vi "Refilderefrescos.vi"() -> ()   [LabVIEW 2020]
uses:
  <vilib>/LabVIEW Interface for Arduino/Type Defs/Board Type.ctl
  <vilib>/LabVIEW Interface for Arduino/Type Defs/Pin Mode.ctl
  <vilib>/LabVIEW Interface for Arduino/LabVIEW Interface for Arduino.lvlib
panel:
  out "Number of bottles made":dbl
  out "¿Lleno?":dbl(slide) scale=0.0..5.0
  out "BomC1":bool
  out "BomC2":bool
  out "BomC3":bool
  out "BomC4":bool
  out "BomT4":bool
  out "BomT3":bool
  out "BomT2":bool
  out "BomT1":bool
  out "Información Adicional":string
  out "Detección":string
  out "Paro":bool
  out "Marcha":bool
  in  "Total Stop":bool
  in  "VISA resource":refnum<visa-resource-name>
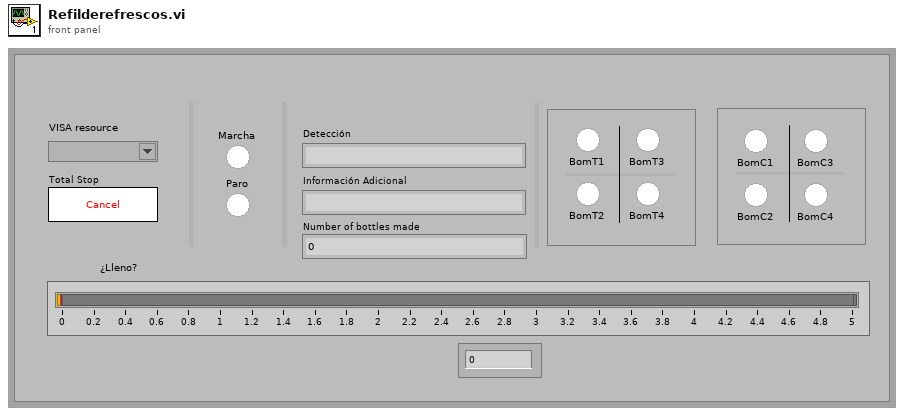
[diagram p1: front panel]
types:
  T1 = typedef "LabVIEW Interface for Arduino.lvlib/Pin Mode.ctl" = enum8{"Input", "Output"}
  T2 = typedef "LabVIEW Interface for Arduino.lvlib/Board Type.ctl" = enum16{"Uno", "Dimuelanove w/Atmega 328", "Mega 2560"}
  T3 = typedef "LabVIEW Interface for Arduino.lvlib/Arduino Resource.ctl" = cluster{"VISA resource":refnum<visa-resource-name>, "Board Type":T2, "Connection Type":enum8{"USB / Serial"}, "Bytes Per Packet (15)":u8}
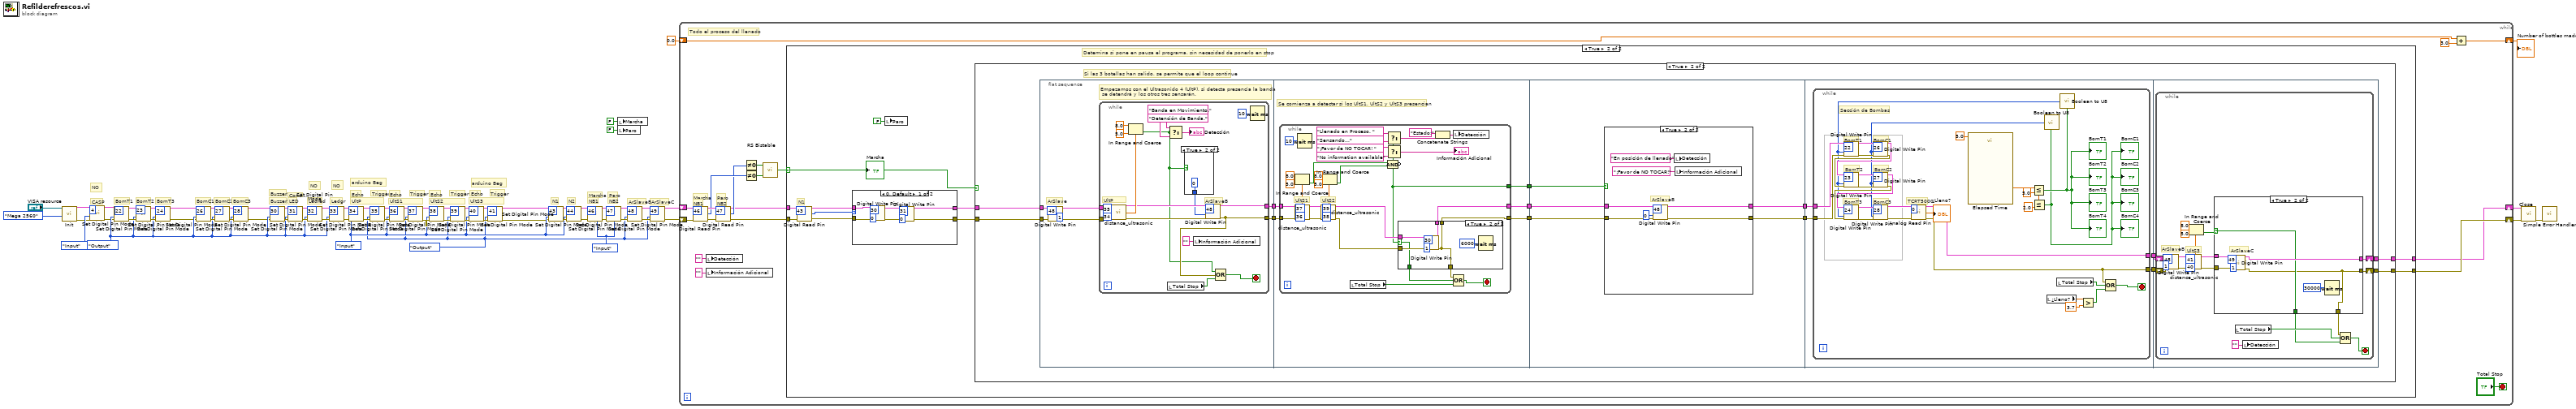
[diagram p0: block diagram]
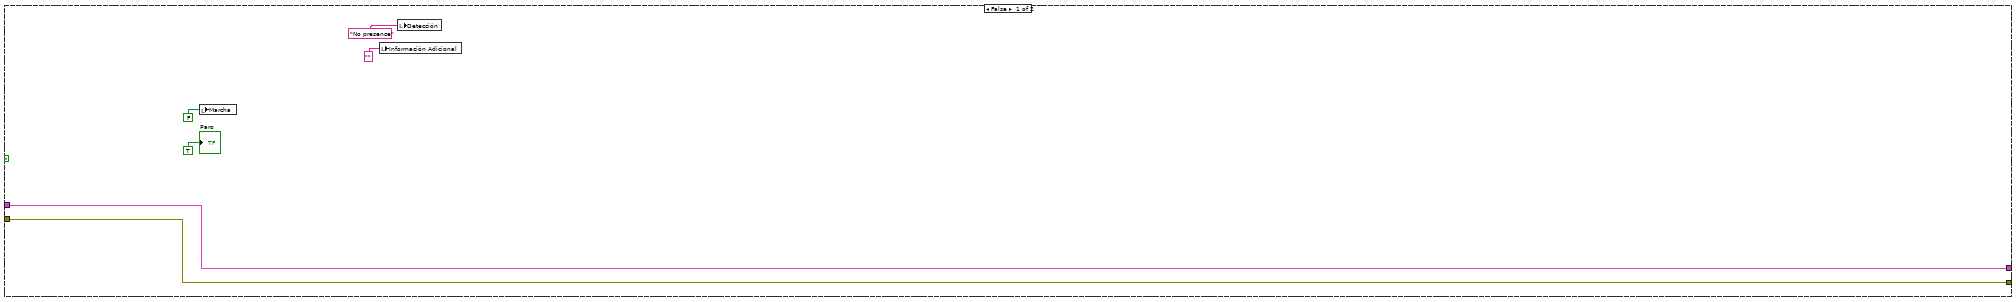
[diagram p2: hidden frame]
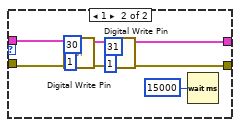
[diagram p3: hidden frame]
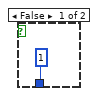
[diagram p5: hidden frame]
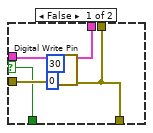
[diagram p6: hidden frame]
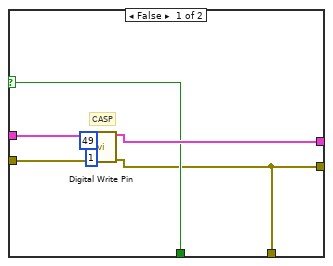
[diagram p8: hidden frame]
diagram:
  w26 = Pin_Mode."Input" ("Pin Mode (Input)")
  w21 = Pin_Mode."Output" ("Pin Mode (Input)")
  w31 = Pin_Mode."Input" ("Pin Mode (Input)")
  w65 = Pin_Mode."Output" ("Pin Mode (Input)")
  # "arduino Beg"
  # "arduino Beg"
  # "NO"
  # "NO"
  # "NO"
  # "Buzzer1"
  # "Condensado"
  # "ArSlaveC"
  # "CASP"
  # "ArSlaveB"
  # "Trigger"
  # "Echo"
  # "Trigger"
  # "Echo"
  # "Trigger"
  # "Echo"
  # "Trigger"
  # "Echo"
  # "Paro"
  # "Marcha"
  # "NB2"
  # "NB1"
  # "N2"
  # "N1"
  # "UltP"
  # "UltS1"
  # "UltS2"
  # "UltS3"
  # "Ledgr"
  # "Ledred"
  # "LED"
  # "Buzzer1"
  # "BomC1"
  # "BomC2"
  # "BomC3"
  # "BomT3"
  # "BomT2"
  # "BomT1"
  n1 = call <vilib>:"Init.vi"("VISA resource"="VISA resource", "Board Type (Uno)"=Board_Type."Mega 2560") -> ("Arduino Resource"=w16:T3, "error out"=w15:errorcluster)  [unwired: 16 in]
  n2 = call <vilib>:"Set Digital Pin Mode.vi"("Arduino Resource"=w16, "Digital I/O Pin"=u8 4, "Pin Mode (Input)"=Pin_Mode."Input", "error in"=w15) -> ("Arduino Resource"=w20:T3, "error out"=w19:errorcluster)  [unwired: 10 in]
  n3 = call <vilib>:"Set Digital Pin Mode.vi"("Arduino Resource"=w20, "Digital I/O Pin"=u8 22, "Pin Mode (Input)"=w65, "error in"=w19) -> ("Arduino Resource"=w89:T3, "error out"=w88:errorcluster)  [unwired: 10 in]
  n4 = call <vilib>:"Set Digital Pin Mode.vi"("Arduino Resource"=w89, "Digital I/O Pin"=u8 23, "Pin Mode (Input)"=w65, "error in"=w88) -> ("Arduino Resource"=w87:T3, "error out"=w86:errorcluster)  [unwired: 10 in]
  n5 = call <vilib>:"Set Digital Pin Mode.vi"("Arduino Resource"=w87, "Digital I/O Pin"=u8 24, "Pin Mode (Input)"=w65, "error in"=w86) -> ("Arduino Resource"=w7:T3, "error out"=w8:errorcluster)  [unwired: 10 in]
  n6 = call <vilib>:"Set Digital Pin Mode.vi"("Arduino Resource"=w7, "Digital I/O Pin"=u8 26, "Pin Mode (Input)"=w65, "error in"=w8) -> ("Arduino Resource"=w85:T3, "error out"=w84:errorcluster)  [unwired: 10 in]
  n7 = call <vilib>:"Set Digital Pin Mode.vi"("Arduino Resource"=w85, "Digital I/O Pin"=u8 27, "Pin Mode (Input)"=w65, "error in"=w84) -> ("Arduino Resource"=w83:T3, "error out"=w82:errorcluster)  [unwired: 10 in]
  n8 = call <vilib>:"Set Digital Pin Mode.vi"("Arduino Resource"=w83, "Digital I/O Pin"=u8 28, "Pin Mode (Input)"=w65, "error in"=w82) -> ("Arduino Resource"=w10:T3, "error out"=w9:errorcluster)  [unwired: 10 in]
  n9 = call <vilib>:"Set Digital Pin Mode.vi"("Arduino Resource"=w10, "Digital I/O Pin"=u8 30, "Pin Mode (Input)"=w65, "error in"=w9) -> ("Arduino Resource"=w69:T3, "error out"=w68:errorcluster)  [unwired: 10 in]
  n10 = call <vilib>:"Set Digital Pin Mode.vi"("Arduino Resource"=w69, "Digital I/O Pin"=u8 31, "Pin Mode (Input)"=w65, "error in"=w68) -> ("Arduino Resource"=w66:T3, "error out"=w67:errorcluster)  [unwired: 10 in]
  n11 = call <vilib>:"Set Digital Pin Mode.vi"("Arduino Resource"=w66, "Digital I/O Pin"=u8 32, "Pin Mode (Input)"=w65, "error in"=w67) -> ("Arduino Resource"=w70:T3, "error out"=w71:errorcluster)  [unwired: 10 in]
  n12 = call <vilib>:"Set Digital Pin Mode.vi"("Arduino Resource"=w70, "Digital I/O Pin"=u8 33, "Pin Mode (Input)"=w65, "error in"=w71) -> ("Arduino Resource"=w74:T3, "error out"=w75:errorcluster)  [unwired: 10 in]
  n13 = call <vilib>:"Set Digital Pin Mode.vi"("Arduino Resource"=w74, "Digital I/O Pin"=u8 34, "Pin Mode (Input)"=w31, "error in"=w75) -> ("Arduino Resource"=w72:T3, "error out"=w73:errorcluster)  [unwired: 10 in]
  n14 = call <vilib>:"Set Digital Pin Mode.vi"("Arduino Resource"=w72, "Digital I/O Pin"=u8 35, "Pin Mode (Input)"=w21, "error in"=w73) -> ("Arduino Resource"=w76:T3, "error out"=w77:errorcluster)  [unwired: 10 in]
  n15 = call <vilib>:"Set Digital Pin Mode.vi"("Arduino Resource"=w76, "Digital I/O Pin"=u8 36, "Pin Mode (Input)"=w31, "error in"=w77) -> ("Arduino Resource"=w78:T3, "error out"=w79:errorcluster)  [unwired: 10 in]
  n16 = call <vilib>:"Set Digital Pin Mode.vi"("Arduino Resource"=w78, "Digital I/O Pin"=u8 37, "Pin Mode (Input)"=w21, "error in"=w79) -> ("Arduino Resource"=w35:T3, "error out"=w36:errorcluster)  [unwired: 10 in]
  n17 = call <vilib>:"Set Digital Pin Mode.vi"("Arduino Resource"=w35, "Digital I/O Pin"=u8 38, "Pin Mode (Input)"=w31, "error in"=w36) -> ("Arduino Resource"=w34:T3, "error out"=w39:errorcluster)  [unwired: 10 in]
  n18 = call <vilib>:"Set Digital Pin Mode.vi"("Arduino Resource"=w34, "Digital I/O Pin"=u8 39, "Pin Mode (Input)"=w21, "error in"=w39) -> ("Arduino Resource"=w33:T3, "error out"=w38:errorcluster)  [unwired: 10 in]
  n19 = call <vilib>:"Set Digital Pin Mode.vi"("Arduino Resource"=w33, "Digital I/O Pin"=u8 40, "Pin Mode (Input)"=w31, "error in"=w38) -> ("Arduino Resource"=w32:T3, "error out"=w37:errorcluster)  [unwired: 10 in]
  n20 = call <vilib>:"Set Digital Pin Mode.vi"("Arduino Resource"=w32, "Digital I/O Pin"=u8 41, "Pin Mode (Input)"=w21, "error in"=w37) -> ("Arduino Resource"=w6:T3, "error out"=w5:errorcluster)  [unwired: 10 in]
  n21 = call <vilib>:"Set Digital Pin Mode.vi"("Arduino Resource"=w6, "Digital I/O Pin"=u8 43, "Pin Mode (Input)"=w31, "error in"=w5) -> ("Arduino Resource"=w80:T3, "error out"=w81:errorcluster)  [unwired: 10 in]
  n22 = call <vilib>:"Set Digital Pin Mode.vi"("Arduino Resource"=w80, "Digital I/O Pin"=u8 44, "Pin Mode (Input)"=w31, "error in"=w81) -> ("Arduino Resource"=w62:T3, "error out"=w63:errorcluster)  [unwired: 10 in]
  n23 = call <vilib>:"Set Digital Pin Mode.vi"("Arduino Resource"=w62, "Digital I/O Pin"=u8 46, "Pin Mode (Input)"=w26, "error in"=w63) -> ("Arduino Resource"=w61:T3, "error out"=w60:errorcluster)  [unwired: 10 in]
  n24 = call <vilib>:"Set Digital Pin Mode.vi"("Arduino Resource"=w61, "Digital I/O Pin"=u8 47, "Pin Mode (Input)"=w26, "error in"=w60) -> ("Arduino Resource"=w29:T3, "error out"=w28:errorcluster)  [unwired: 10 in]
  n25 = local write "Marcha"(FALSE ("Marcha")) -> ()
  n26 = local write "Paro"(FALSE ("Paro")) -> ()
  n27 = call <vilib>:"Set Digital Pin Mode.vi"("Arduino Resource"=w29, "Digital I/O Pin"=u8 48, "Pin Mode (Input)"=w21, "error in"=w28) -> ("Arduino Resource"=w25:T3, "error out"=w24:errorcluster)  [unwired: 10 in]
  n28 = call <vilib>:"Set Digital Pin Mode.vi"("Arduino Resource"=w25, "Digital I/O Pin"=u8 49, "Pin Mode (Input)"=w21, "error in"=w24) -> ("Arduino Resource"=w23:T3, "error out"=w1:errorcluster)  [unwired: 10 in]
  n29 = while {
    shift-right: [w100] -> w14
    shift-left: 0.0 -> [w98]
    shift-right: [w95] -> w2
    shift-left: w23 -> [w112]
    shift-right: [w96] -> w13
    shift-left: w1 -> [w94]
    stop <- "Total Stop" stop-if-true
    # "Marcha"
    # "NB1"
    # "Paro"
    # "NB2"
    # "Todo el proceso del llenado"
    n30 = call <vilib>:"Digital Read Pin.vi"("Arduino Resource"=w112, "Digital I/O Pin (0)"=u8 46, "error in"=w94) -> ("Arduino Resource"=w108:T3, "Value"=w107:u8, "error out"=w109:errorcluster)  [unwired: 10 in]
    n31 = local write "Detección"("" ("Detección")) -> ()
    n32 = local write "Información Adicional"("" ("Información Adicional")) -> ()
    n33 = call <vilib>:"Digital Read Pin.vi"("Arduino Resource"=w108, "Digital I/O Pin (0)"=u8 47, "error in"=w109) -> ("Arduino Resource"=w102:T3, "Value"=w106:u8, "error out"=w101:errorcluster)  [unwired: 10 in]
    n34 = Not Equal To 0?(x=w106) -> (x != 0?=w105:bool)
    n35 = Not Equal To 0?(x=w107) -> (x != 0?=w104:bool)
    n36 = call "RS Bistable.vi"("Set"=w104, "Reset"=w105) -> ("Salida (Q)"=w103:bool)
    n37 = case shown="True" w103 {
      selector: w103 -> [_ w128]
      tunnel: w102 -> [w116 w127]
      tunnel: w101 -> [w115 w126]
      tunnel: [w115 w130] -> w96
      tunnel: [w116 w129] -> w95
      frame False {
        n38 = local write "Marcha"(FALSE ("Marcha")) -> ()
        n39 = local write "Información Adicional"("" ("Información Adicional")) -> ()
        n40 = local write "Detección"("No presence" ("Detección")) -> ()
        "Paro" <- TRUE ("Paro")
      }
      frame True {
        # "N1"
        # "Detemina si pone en pausa el programa, sin necesidad de ponerlo en stop"
        n41 = call <vilib>:"Digital Read Pin.vi"("Arduino Resource"=w127, "Digital I/O Pin (0)"=u8 43, "error in"=w126) -> ("Arduino Resource"=w123:T3, "Value"=w124:u8, "error out"=w122:errorcluster)  [unwired: 10 in]
        n42 = case shown="0, Default" w124 {
          tunnel: w123 -> [w138 w148]
          tunnel: w122 -> [w137 w147]
          tunnel: [w132 w141] -> w121
          tunnel: [w131 w142] -> w120
          frame 0, Default {
            n43 = call <vilib>:"Digital Write Pin.vi"("Arduino Resource"=w138, "Digital I/O Pin (0)"=u8 30, "Value (0)"=u8 0, "error in"=w137) -> ("Arduino Resource"=w134:T3, "error out"=w133:errorcluster)  [unwired: 10 in]
            n44 = call <vilib>:"Digital Write Pin.vi"("Arduino Resource"=w134, "Digital I/O Pin (0)"=u8 31, "Value (0)"=u8 0, "error in"=w133) -> ("Arduino Resource"=w131:T3, "error out"=w132:errorcluster)  [unwired: 10 in]
          }
          frame 1 {
            n45 = call <vilib>:"Digital Write Pin.vi"("Arduino Resource"=w148, "Digital I/O Pin (0)"=u8 30, "Value (0)"=u8 1, "error in"=w147) -> ("Arduino Resource"=w143:T3, "error out"=w144:errorcluster)  [unwired: 10 in]
            n46 = call <vilib>:"Digital Write Pin.vi"("Arduino Resource"=w143, "Digital I/O Pin (0)"=u8 31, "Value (0)"=u8 1, "error in"=w144) -> ("Arduino Resource"=w142:T3, "error out"=w141:errorcluster)  [unwired: 10 in]
            n47 = Wait (ms)(milliseconds to wait=u32 15000) -> ()  [unwired: 1 out]
          }
        }
        n48 = local write "Paro"(FALSE ("Paro")) -> ()
        n49 = case shown="True" w128 {
          tunnel: w120 -> [w152 w164]
          tunnel: w121 -> [w153 w163]
          tunnel: [w153 w155] -> w130
          tunnel: [w152 w154] -> w129
          frame False {
          }
          frame True {
            # "Si las 3 botellas han salido, se permite que el loop continue"
            n50 = flat-sequence {
              tunnel: w164 -> [w172]
              tunnel: w163 -> [w171]
              tunnel: [w174] -> w166
              tunnel: [w173] -> w165
              tunnel: w166 -> [w202]
              tunnel: w165 -> [w201]
              tunnel: [w200] -> w160
              tunnel: [w199] -> w158
              tunnel: [w198] -> w156
              tunnel: w160 -> [w256]
              tunnel: [w252] -> w159
              tunnel: w158 -> [w255]
              tunnel: [w253] -> w157
              tunnel: w156 -> [w254]
              tunnel: w159 -> [w270]
              tunnel: w157 -> [w269]
              tunnel: [w268] -> w162
              tunnel: [w267] -> w161
              tunnel: w162 -> [w310]
              tunnel: w161 -> [w311]
              tunnel: [w309] -> w155
              tunnel: [w308] -> w154
              frame #0 {
                # "ArSlave"
                # "Empezamos con el Ultrasonido 4 (UltP), si detecta presencia la banda\n se detendrá y los otros tres sensarán."
                n51 = call <vilib>:"Digital Write Pin.vi"("Arduino Resource"=w172, "Digital I/O Pin (0)"=u8 48, "Value (0)"=u8 1, "error in"=w171) -> ("Arduino Resource"=w169:T3, "error out"=w170:errorcluster)  [unwired: 10 in]
                n52 = while {
                  tunnel: w169 -> [w195]
                  tunnel: w170 -> [w194]
                  tunnel: [w177] -> w174
                  tunnel: [w182] -> w173
                  stop <- w191 stop-if-true
                  # "ArSlaveB"
                  # "UltP"
                  n53 = call <vilib>:"distance_ultrasonic.vi"("Arduino Resource"=w195, "Trigger"=u8 35, "Echo"=u8 34, "error in"=w194) -> ("Arduino Resource"=w181:T3, "Distance(cm)"=w189:dbl, "error out"=w178:errorcluster)  [unwired: 9 in]
                  n54 = In Range and Coerce(upper limit=8.0, x=w189, lower limit=5.0) -> (In Range?=w176:bool)  [unwired: 1 out]
                  n55 = local read "Total Stop"() -> (w175:bool)
                  n56 = Select(t="Detención de Banda.", s=w176, f="Banda en Movimiento.") -> (s? t:f=→"Detección":string)
                  n57 = case shown="True" w176 {
                    tunnel: [u8 1 u8 0] -> w179
                    frame False {
                    }
                    frame True {
                    }
                  }
                  n58 = local write "Información Adicional"("" ("Información Adicional")) -> ()
                  n59 = call <vilib>:"Digital Write Pin.vi"("Arduino Resource"=w181, "Digital I/O Pin (0)"=u8 48, "Value (0)"=w179, "error in"=w178) -> ("Arduino Resource"=w182:T3, "error out"=w177:errorcluster)  [unwired: 10 in]
                  n60 = Compound Arithmetic op=OR(w176, w177, w175) -> (w191:bool)
                  n61 = Wait (ms)(milliseconds to wait=u32 10) -> ()  [unwired: 1 out]
                }
              }
              frame #1 {
                # "Se comienza a detectar si los UltS1, UltS2 y UltS3 presencian"
                n62 = while {
                  tunnel: w202 -> [w228]
                  tunnel: w201 -> [w227]
                  tunnel: [w207] -> w200
                  tunnel: [w206] -> w199
                  tunnel: [w205] -> w198
                  stop <- w236 stop-if-true
                  # "UltS2"
                  # "UltS1"
                  n63 = call <vilib>:"distance_ultrasonic.vi"("Arduino Resource"=w227, "Trigger"=u8 37, "Echo"=u8 36, "error in"=w228) -> ("Arduino Resource"=w229:T3, "Distance(cm)"=w224:dbl, "error out"=w230:errorcluster)  [unwired: 9 in]
                  n64 = In Range and Coerce(upper limit=8.0, x=w224, lower limit=5.0) -> (In Range?=w219:bool)  [unwired: 1 out]
                  n65 = Wait (ms)(milliseconds to wait=u32 10) -> ()  [unwired: 1 out]
                  n66 = call <vilib>:"distance_ultrasonic.vi"("Arduino Resource"=w229, "Trigger"=u8 39, "Echo"=u8 38, "error in"=w230) -> ("Arduino Resource"=w209:T3, "Distance(cm)"=w221:dbl, "error out"=w208:errorcluster)  [unwired: 9 in]
                  n67 = In Range and Coerce(upper limit=8.0, x=w221, lower limit=5.0) -> (In Range?=w220:bool)  [unwired: 1 out]
                  n68 = local read "Total Stop"() -> (w235:bool)
                  n69 = Compound Arithmetic op=AND(w219, w220) -> (invert w205:bool)
                  n70 = Select(t="Llenado en Proceso. ", s=w205, f="Sensando...") -> (s? t:f=w210:string)
                  n71 = Select(t="¡Favor de NO TOCAR! ", s=w205, f="No information available") -> (s? t:f=→"Información Adicional":string)
                  n72 = case shown="True" w205 {
                    selector: w205 -> [w238 w245]
                    tunnel: w209 -> [w241 w251]
                    tunnel: w208 -> [w240 w248]
                    tunnel: [w237 w244] -> w207
                    tunnel: [w239 w246] -> w206
                    tunnel: [w238 w245] -> w204
                    tunnel: [w237 w244] -> w203
                    frame False {
                      n73 = call <vilib>:"Digital Write Pin.vi"("Arduino Resource"=w241, "Digital I/O Pin (0)"=u8 30, "Value (0)"=u8 0, "error in"=w240) -> ("Arduino Resource"=w239:T3, "error out"=w237:errorcluster)  [unwired: 10 in]
                    }
                    frame True {
                      n74 = call <vilib>:"Digital Write Pin.vi"("Arduino Resource"=w251, "Digital I/O Pin (0)"=u8 30, "Value (0)"=u8 1, "error in"=w248) -> ("Arduino Resource"=w246:T3, "error out"=w244:errorcluster)  [unwired: 10 in]
                      n75 = Wait (ms)(milliseconds to wait=u32 6000) -> ()  [unwired: 1 out]
                    }
                  }
                  n76 = Concatenate Strings("Estado:" ("string"), w210) -> (w211:string)
                  n77 = Compound Arithmetic op=OR(w203, w204, w235) -> (w236:bool)
                  n78 = local write "Detección"(w211) -> ()
                }
              }
              frame #2 {
                n79 = case shown="True" w254 {
                  tunnel: w256 -> [w257 w266]
                  tunnel: w255 -> [w258 w265]
                  tunnel: [w258 w262] -> w253
                  tunnel: [w257 w259] -> w252
                  frame False {
                  }
                  frame True {
                    # "ArSlaveB"
                    n80 = call <vilib>:"Digital Write Pin.vi"("Arduino Resource"=w265, "Digital I/O Pin (0)"=u8 48, "Value (0)"=u8 0, "error in"=w266) -> ("Arduino Resource"=w262:T3, "error out"=w259:errorcluster)  [unwired: 10 in]
                    n81 = local write "Detección"("En posición de llenado" ("Detección")) -> ()
                    n82 = local write "Información Adicional"("¡Favor de NO TOCAR!" ("Información Adicional")) -> ()
                  }
                }
              }
              frame #3 {
                n83 = while {
                  tunnel: w270 -> [w307]
                  tunnel: w269 -> [w305]
                  tunnel: [w271] -> w267
                  tunnel: [w280] -> w268
                  stop <- w303 stop-if-true
                  # "TCRT5000"
                  # "BomC1"
                  # "BomC2"
                  # "BomC3"
                  # "BomT3"
                  # "BomT2"
                  # "BomT1"
                  # "Sección de Bombas"
                  n84 = call "Elapsed Time"("Time Target (s)"=5.0) -> ("Elapsed Time (s)"=w292:dbl)  [unwired: 11 in, 7 out]
                  n85 = Less Or Equal?(x=w292, y=5.0) -> (x <= y?=w291:bool)
                  "BomT1" <- w291
                  "BomT2" <- w291
                  "BomT3" <- w291
                  "BomT4" <- w291
                  n86 = Less Or Equal?(x=w292, y=2.0) -> (x <= y?=w290:bool)
                  "BomC1" <- w290
                  "BomC2" <- w290
                  "BomC3" <- w290
                  "BomC4" <- w290
                  n87 = call "Boolean to U8.vi"("?1=0"=w290) -> ("U8"=w288:u8)
                  n88 = local read "¿Lleno?"() -> (w277:dbl)
                  n89 = local read "Total Stop"() -> (w278:bool)
                  n90 = call "Boolean to U8.vi"("?1=0"=w291) -> ("U8"=w289:u8)
                  n91 = call <vilib>:"Digital Write Pin.vi"("Arduino Resource"=w305, "Digital I/O Pin (0)"=u8 22, "Value (0)"=w289, "error in"=w307) -> ("Arduino Resource"=w304:T3, "error out"=w306:errorcluster)  [unwired: 10 in]
                  n92 = call <vilib>:"Digital Write Pin.vi"("Arduino Resource"=w304, "Digital I/O Pin (0)"=u8 26, "Value (0)"=w288, "error in"=w306) -> ("Arduino Resource"=w300:T3, "error out"=w299:errorcluster)  [unwired: 10 in]
                  n93 = call <vilib>:"Digital Write Pin.vi"("Arduino Resource"=w300, "Digital I/O Pin (0)"=u8 23, "Value (0)"=w289, "error in"=w299) -> ("Arduino Resource"=w302:T3, "error out"=w301:errorcluster)  [unwired: 10 in]
                  n94 = call <vilib>:"Digital Write Pin.vi"("Arduino Resource"=w302, "Digital I/O Pin (0)"=u8 27, "Value (0)"=w288, "error in"=w301) -> ("Arduino Resource"=w295:T3, "error out"=w296:errorcluster)  [unwired: 10 in]
                  n95 = call <vilib>:"Digital Write Pin.vi"("Arduino Resource"=w295, "Digital I/O Pin (0)"=u8 24, "Value (0)"=w289, "error in"=w296) -> ("Arduino Resource"=w297:T3, "error out"=w298:errorcluster)  [unwired: 10 in]
                  n96 = call <vilib>:"Digital Write Pin.vi"("Arduino Resource"=w297, "Digital I/O Pin (0)"=u8 28, "Value (0)"=w288, "error in"=w298) -> ("Arduino Resource"=w273:T3, "error out"=w272:errorcluster)  [unwired: 10 in]
                  n97 = call <vilib>:"Analog Read Pin.vi"("Arduino Resource"=w273, "Analog Input Pin (0)"=u8 0, "error in"=w272) -> ("Arduino Resource"=w280:T3, "Voltage"=→"¿Lleno?":dbl, "error out"=w271:errorcluster)  [unwired: 10 in]
                  n98 = Greater?(x=w277, y=3.7) -> (0:w275:bool)
                  n99 = Compound Arithmetic op=OR(w271, w278, w275) -> (w303:bool)
                }
              }
              frame #4 {
                n100 = while {
                  shift-right: [w318] -> w309
                  shift-left: w311 -> [w329]
                  shift-right: [w317] -> w308
                  shift-left: w310 -> [w328]
                  stop <- w314 stop-if-true
                  # "UltS3"
                  # "ArSlaveB"
                  n101 = call <vilib>:"Digital Write Pin.vi"("Arduino Resource"=w328, "Digital I/O Pin (0)"=u8 48, "Value (0)"=u8 1, "error in"=w329) -> ("Arduino Resource"=w323:T3, "error out"=w322:errorcluster)  [unwired: 10 in]
                  n102 = call <vilib>:"distance_ultrasonic.vi"("Arduino Resource"=w323, "Trigger"=u8 41, "Echo"=u8 40, "error in"=w322) -> ("Arduino Resource"=w319:T3, "Distance(cm)"=w324:dbl, "error out"=w320:errorcluster)  [unwired: 9 in]
                  n103 = In Range and Coerce(upper limit=8.0, x=w324, lower limit=5.0) -> (In Range?=w321:bool)  [unwired: 1 out]
                  n104 = case shown="True" w321 {
                    selector: w321 -> [w334 w341]
                    tunnel: w320 -> [w337 w347]
                    tunnel: w319 -> [w338 w346]
                    tunnel: [w333 w340] -> w318
                    tunnel: [w335 w345] -> w317
                    tunnel: [w334 w341] -> w313
                    tunnel: [w333 w340] -> w312
                    frame False {
                      # "CASP"
                      n105 = call <vilib>:"Digital Write Pin.vi"("Arduino Resource"=w338, "Digital I/O Pin (0)"=u8 49, "Value (0)"=u8 1, "error in"=w337) -> ("Arduino Resource"=w335:T3, "error out"=w333:errorcluster)  [unwired: 10 in]
                    }
                    frame True {
                      # "ArSlaveC"
                      n106 = call <vilib>:"Digital Write Pin.vi"("Arduino Resource"=w346, "Digital I/O Pin (0)"=u8 49, "Value (0)"=u8 1, "error in"=w347) -> ("Arduino Resource"=w345:T3, "error out"=w340:errorcluster)  [unwired: 10 in]
                      n107 = Wait (ms)(milliseconds to wait=u32 30000) -> ()  [unwired: 1 out]
                    }
                  }
                  n108 = local read "Total Stop"() -> (w315:bool)
                  n109 = local write "Detección"("" ("Detección")) -> ()
                  n110 = Compound Arithmetic op=OR(w312, w315, w313) -> (w314:bool)
                }
              }
            }
          }
        }
        "Marcha" <- w128
      }
    }
    n111 = Add(x=w98, y=3.0) -> (x+y=w100:dbl)
  }
  "Number of bottles made" <- w14
  n112 = call <vilib>:"Close.vi"("Arduino Resource"=w2, "error in"=w13) -> ("error out"=w12:errorcluster)  [unwired: 13 in]
  n113 = call <vilib>:"Simple Error Handler.vi"("error in (no error)"=w12) -> ()  [unwired: 4 in, 5 out]
